vi "gSEL.vi"() -> ()   [LabVIEW 2011]
panel:
  in  "gSEL":i32
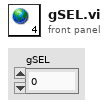
[diagram p1: front panel]
diagram:
